vi "Sub_Build_Variable_Header_Connect.vi"(8 "error in (no error)":errorcluster, 11 "Authenticate":bool) -> (0 "error out":errorcluster, 2 "Variable Header":u8[](array[numeric]) format="%x")   [LabVIEW 2013, in "IOTFoundation.lvlib"]
uses:
  IOTFoundation.lvlib
panel:
  in  "Protocol Name":string="MQIsdp"
  in  "Protocol Version":u8=3
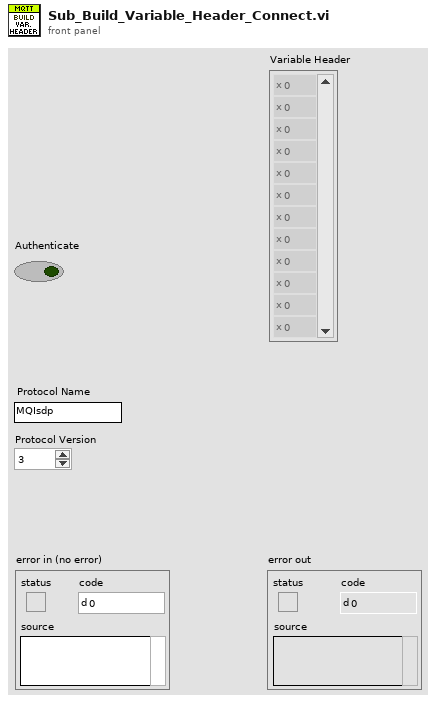
[diagram p1: front panel]
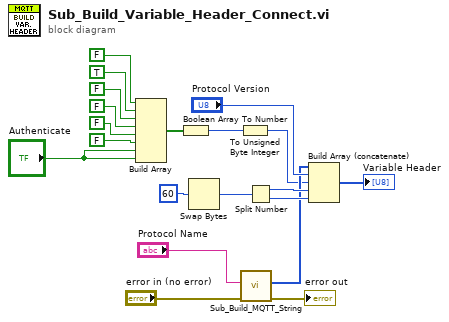
[diagram p0: block diagram]
diagram:
  n1 = Build Array(FALSE, TRUE, FALSE, FALSE, FALSE, FALSE, "Authenticate", "Authenticate") -> (w4:bool[])
  n2 = Boolean Array To Number(Boolean array=w4) -> (number=w11:u32)
  n3 = Swap Bytes(anything=60) -> (byte swapped=w20:i32)
  n4 = To Unsigned Byte Integer(number=w11) -> (unsigned 8bit integer=w3:u8)
  n5 = call "Sub_Build_MQTT_String.vi"("error in (no error)"="error in (no error)", "String to be encoded"="Protocol Name") -> ("error out"=→"error out":errorcluster, "UTF8 Byte Array"=w14:u8[])  [unwired: 8 in]
  n6 = Split Number(x=w20) -> (hi(x)=w19:u16, lo(x)=w18:u16)
  n7 = Build Array (concatenate)(w14, "Protocol Version", w3, w19, w18) -> (→"Variable Header":u16[])
